vi "DWA Array to Register to Write Array.vi"(8 "error in (no error)":errorcluster, 11 "Toggle 7.1 in":refnum<class "Toggle 7.1.lvclass">) -> (0 "error out":errorcluster, 1 "DWA Values":dbl[](array[numeric]), 2 "DWA Settings":T1[](array[typedef]), 3 "Toggle 7.1 out":refnum<class "Toggle 7.1.lvclass">)   [LabVIEW 2020, in "Toggle 7.1.lvclass"]
doc: "Getting the Charge pump array and makes it into registers"
uses:
  Toggle 7.1.lvclass
  Controls/Register to Write.ctl
  Toggle 7.1.lvclass/Toggle 7.1.ctl
  PIC-device/PIC-Device.lvclass
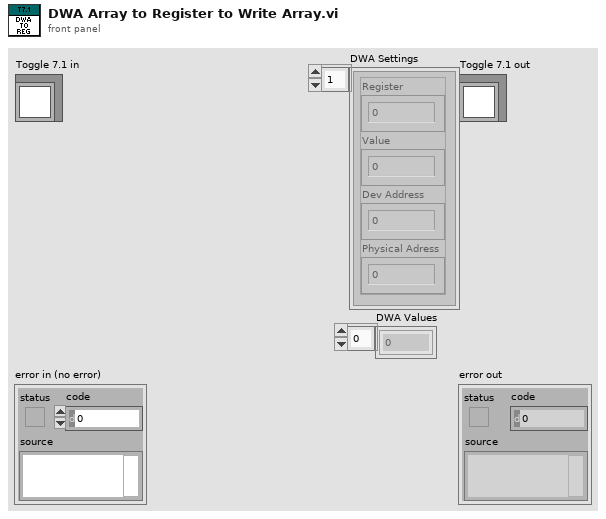
[diagram p1: front panel]
types:
  T1 = typedef "PIC-Device.lvclass/Register to Write.ctl" = cluster{"Register":u32, "Value":u32, "Dev Address":u32, "Physical Adress":u32}
  T2 = typedef "Toggle 7.1.lvclass/Parameter Cluster.ctl" = cluster{"Enable":bool, "Register Number":u32, "Use Array":bool, "Array":dbl[], "To From Cluster":cluster{"From":dbl, "To":dbl, "Step":dbl}}
  T3 = typedef "Toggle 7.1.lvclass/Charge Pump Information cluster.ctl" = cluster{"Min":dbl, "Max":dbl, "Step":dbl, "Default":dbl}
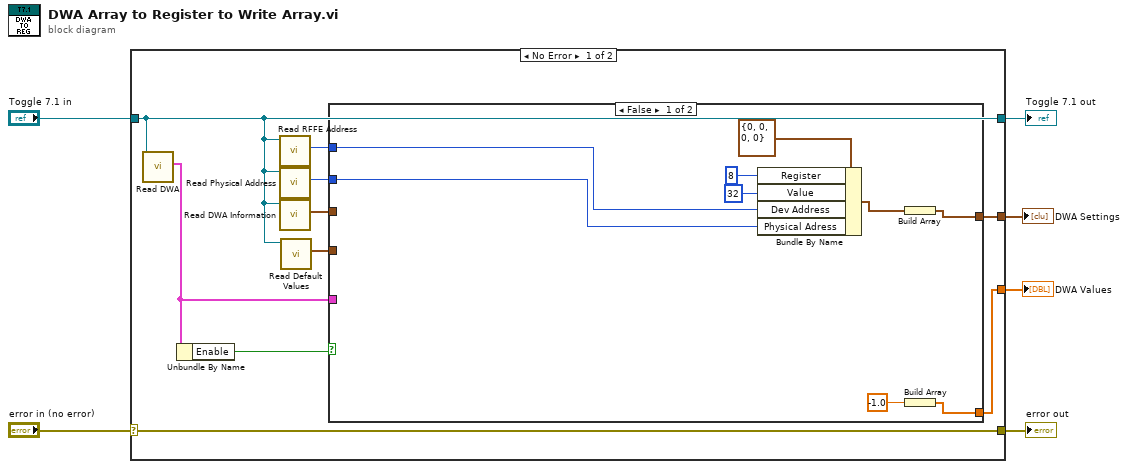
[diagram p0: block diagram]
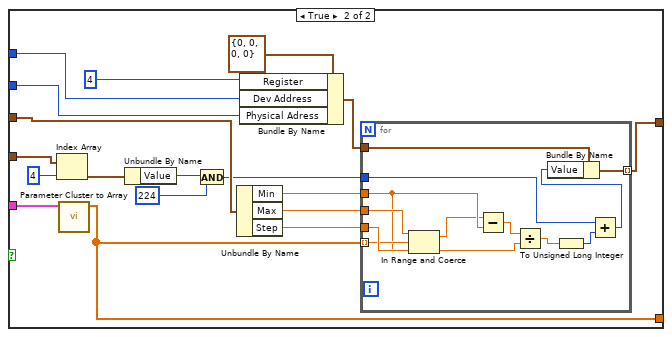
[diagram p2: hidden frame]
diagram:
  n1 = case shown="No Error" "error in (no error)" {
    selector: "error in (no error)" -> [w16 w57]
    tunnel: [w16 w57] -> w5
    tunnel: [w8 w56] -> w3
    tunnel: "Toggle 7.1 in" -> [w8 w56]
    tunnel: [w15 _] -> w2
    tunnel: [w13 _] -> w1
    frame No Error {
      n2 = call "Read DWA.vi"("Toggle 7.1 in"=w8) -> ("Parameter Cluster"=w14:T2)  [unwired: 9 in, 1 out]
      n3 = Unbundle By Name(w14) -> ("Enable"=w9:bool)
      n4 = call-dynamic "Read RFFE Address.vi"("Toggle 6 in"=w8) -> ("RFFE Adress"=w12:u32)  [unwired: 8 in, 2 out]
      n5 = call-dynamic "Read Physical Address.vi"("Toggle 6 in"=w8) -> ("Physical Adress"=w11:u32)  [unwired: 9 in, 1 out]
      n6 = call "Read DWA Information.vi"("Toggle 7.1 in"=w8) -> ("DWA Information"=w10:T3)  [unwired: 9 in, 1 out]
      n7 = call-dynamic "Read Default Values.vi"("Toggle 7.1 in"=w8) -> ("Default Values"=w7:T1[])  [unwired: 9 in, 1 out]
      n8 = case shown="False" w9 {
        tunnel: [w19 w43] -> w15
        tunnel: w14 -> [_ w42]
        tunnel: [w17 w41] -> w13
        tunnel: w12 -> [w22 w38]
        tunnel: w11 -> [w21 w37]
        tunnel: w10 -> [_ w35]
        tunnel: w7 -> [_ w31]
        frame False {
          n9 = Bundle By Name(cluster=T1 {"Register"=0, "Value"=0, "Dev Address"=0, "Physical Adress"=0} ("Register to Write"), "Register"=u32 8, "Value"=u32 32, "Dev Address"=w22, "Physical Adress"=w21) -> (w20:T1)
          n10 = Build Array(w20) -> (w19:T1[])
          n11 = Build Array(-1.0 ("element")) -> (w17:dbl[])
        }
        frame True {
          n12 = Index Array(array=w31, index=4) -> (element=w29:T1)
          n13 = call "Parameter Cluster to Array.vi"("Parameter Cluster"=w42) -> ("Array"=w41:dbl[])  [unwired: 10 in]
          n14 = Unbundle By Name(w29) -> ("Value"=w28:u32)
          n15 = And(x=w28, y=u32 224) -> (x .and. y?=w26:u32)
          n16 = Unbundle By Name(w35) -> ("Min"=w34:dbl, "Max"=w33:dbl, "Step"=w32:dbl)
          n17 = Bundle By Name(cluster=T1 {"Register"=0, "Value"=0, "Dev Address"=0, "Physical Adress"=0} ("Register to Write"), "Register"=u32 4, "Dev Address"=w38, "Physical Adress"=w37) -> (w36:T1)
          n18 = for {
            tunnel: w36 -> [w55]
            tunnel: w41 -> [w52] mode=indexing
            tunnel: w34 -> [w50]
            tunnel: w33 -> [w51]
            tunnel: w32 -> [w53]
            tunnel: [w47] -> w43 mode=indexing
            tunnel: w26 -> [w44]
            n19 = In Range and Coerce(upper limit=w51, x=w52, lower limit=w50) -> (coerced(x)=w49:dbl)  [unwired: 1 out]
            n20 = Subtract(x=w49, y=w50) -> (x-y=w54:dbl)
            n21 = Divide(x=w54, y=w53) -> (x/y=w48:dbl)
            n22 = To Unsigned Long Integer(number=w48) -> (unsigned 32bit integer=w46:u32)
            n23 = Add(x=w44, y=w46) -> (x+y=w45:u32)
            n24 = Bundle By Name(cluster=w55, "Value"=w45) -> (w47:T1)
          }
        }
      }
    }
    frame Error {
    }
  }
  "error out" <- w5
  "Toggle 7.1 out" <- w3
  "DWA Settings" <- w2
  "DWA Values" <- w1
